vi "test-timer-rollover.vi"() -> ()   [LabVIEW 2019]
uses:
  <vilib>/Rock Robotics/WPI/ThirdParty/JAS_Junk/TrajLib/Trajectory_Library.lvlib
panel:
  out "T2 End":bool
  out "T2 Started":bool
  out "T1 End":bool
  out "T1 Started":bool
  out "T0 Done":bool
  out "Loop 3":i32
  out "Loop 2":i32
  out "Loop 1":i32
  out "rollover 2":i32 format="%36.0f"
  out "T2 - Diff = 4500 good":dbl
  out "T2 - Diff = 4500 no roll":dbl
  out "T0 - Diff = 10 good":dbl
  out "T0 - Diff = 10 no roll":dbl
  out "rollover end":i32 format="%36.0f"
  out "rollover start":i32 format="%36.0f"
  out "T1 - Diff = 4500 good":dbl
  out "T1 - Diff = 4500 no roll":dbl
  # "Get FPGA time.   Test rollover protection."
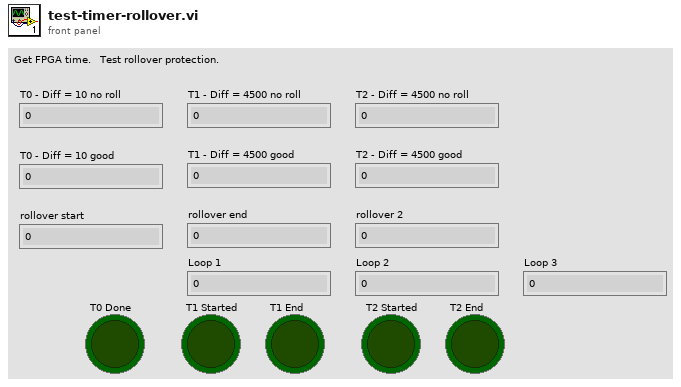
[diagram p1: front panel]
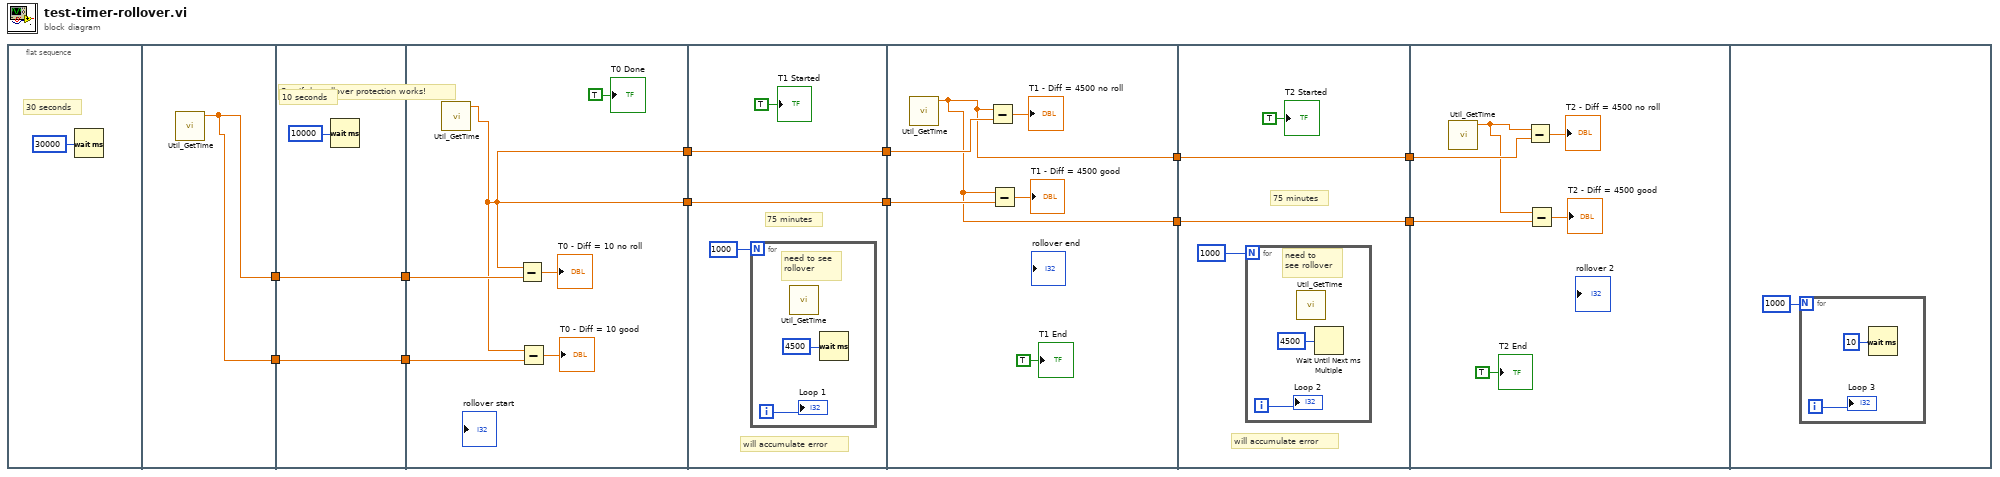
[diagram p0: block diagram]
diagram:
  # "See if the rollover protection works!"
  n1 = flat-sequence {
    tunnel: [w14] -> w8
    tunnel: [w14] -> w6
    tunnel: w8 -> [w16]
    tunnel: [w16] -> w7
    tunnel: w6 -> [w15]
    tunnel: [w15] -> w5
    tunnel: [w18] -> w11
    tunnel: [w18] -> w10
    tunnel: w7 -> [w21]
    tunnel: w5 -> [w20]
    tunnel: [w27] -> w12
    tunnel: w11 -> [w27]
    tunnel: w10 -> [w26]
    tunnel: [w26] -> w9
    tunnel: w12 -> [w35]
    tunnel: w9 -> [w32]
    tunnel: [w30] -> w4
    tunnel: [w30] -> w2
    tunnel: w4 -> [w39]
    tunnel: [w39] -> w3
    tunnel: w2 -> [w38]
    tunnel: [w38] -> w1
    tunnel: w3 -> [w45]
    tunnel: w1 -> [w44]
    frame #0 {
      # "30 seconds"
      n2 = Wait (ms)(milliseconds to wait=u32 30000) -> ()  [unwired: 1 out]
    }
    frame #1 {
      n3 = call <vilib>:"Util_GetTime.vi"() -> ("FPGA_Time_Seconds"=w14:dbl)  [unwired: 11 in]
    }
    frame #2 {
      # "10 seconds"
      n4 = Wait (ms)(milliseconds to wait=u32 10000) -> ()  [unwired: 1 out]
    }
    frame #3 {
      n5 = call <vilib>:"Util_GetTime.vi"() -> ("FPGA_Time_Seconds"=w18:dbl)  [unwired: 11 in]
      n6 = Subtract(x=w18, y=w21) -> (x-y=→"T0 - Diff = 10 no roll":dbl)
      n7 = Subtract(x=w18, y=w20) -> (x-y=→"T0 - Diff = 10 good":dbl)
      "T0 Done" <- TRUE ("T0 Done")
    }
    frame #4 {
      # "will accumulate error"
      # "75 minutes"
      n8 = for {
        N: 1000 -> [_]
        i -> [w28]
        # "need to see\nrollover"
        n9 = call <vilib>:"Util_GetTime.vi"() -> ()  [unwired: 11 in, 1 out]
        n10 = Wait (ms)(milliseconds to wait=u32 4500) -> ()  [unwired: 1 out]
        "Loop 1" <- w28
      }
      "T1 Started" <- TRUE ("T1 Started")
    }
    frame #5 {
      n11 = call <vilib>:"Util_GetTime.vi"() -> ("FPGA_Time_Seconds"=w30:dbl)  [unwired: 11 in]
      n12 = Subtract(x=w30, y=w35) -> (x-y=→"T1 - Diff = 4500 no roll":dbl)
      n13 = Subtract(x=w30, y=w32) -> (x-y=→"T1 - Diff = 4500 good":dbl)
      "T1 End" <- TRUE ("T1 End")
    }
    frame #6 {
      # "will accumulate error"
      # "75 minutes"
      n14 = for {
        N: 1000 -> [_]
        i -> [w40]
        # "need to \nsee rollover"
        n15 = call <vilib>:"Util_GetTime.vi"() -> ()  [unwired: 11 in, 1 out]
        n16 = Wait Until Next ms Multiple(millisecond multiple=u32 4500 ("milliseconds to wait")) -> ()  [unwired: 1 out]
        "Loop 2" <- w40
      }
      "T2 Started" <- TRUE ("T2 Started")
    }
    frame #7 {
      n17 = call <vilib>:"Util_GetTime.vi"() -> ("FPGA_Time_Seconds"=w42:dbl)  [unwired: 11 in]
      n18 = Subtract(x=w42, y=w45) -> (x-y=→"T2 - Diff = 4500 no roll":dbl)
      n19 = Subtract(x=w42, y=w44) -> (x-y=→"T2 - Diff = 4500 good":dbl)
      "T2 End" <- TRUE ("T2 End")
    }
    frame #8 {
      n20 = for {
        N: 1000 -> [_]
        i -> [w49]
        n21 = Wait (ms)(milliseconds to wait=u32 10) -> ()  [unwired: 1 out]
        "Loop 3" <- w49
      }
    }
  }
